vi "Load Fake Flag.vi"(7 "section":string, 8 "error in (no error)":errorcluster, 11 "config ref in":T1) -> (0 "error out":errorcluster, 2 "Fake":bool, 4 "config ref out":T1)   [LabVIEW 2013]
uses:
  <vilib>/Utility/config.llb/Config Data RefNum.ctl
  <vilib>/Utility/config.llb/Read Key (Boolean).vi
  <vilib>/Utility/config.llb/NI_LVConfig.lvlib
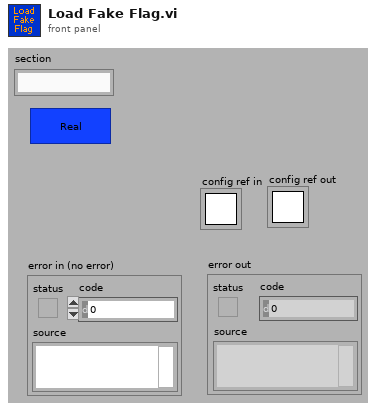
[diagram p1: front panel]
types:
  T1 = typedef "NI_LVConfig.lvlib/Config Data RefNum.ctl" = refnum<k1>
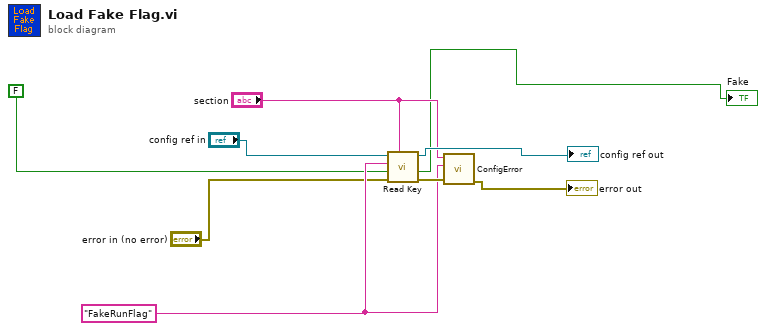
[diagram p0: block diagram]
diagram:
  w5 = "FakeRunFlag" ("key")
  n1 = call-poly <vilib>:"Read Key.vi"("section"="section", "error in (no error)"="error in (no error)", "default value"=FALSE ("2 LBCB Archiving Mode"), "key"=w5, "refnum"="config ref in") -> ("error out"=w9:errorcluster, "value"=→"Fake":bool, "refnum out"=→"config ref out":T1)  [unwired: 3 in, 1 out]
  n2 = call "ConfigError.vi"("error in (no error)"=w9, "Key"=w5, "Section"="section") -> ("error out"=→"error out":errorcluster)  [unwired: 8 in]
